vi "myRIO_BRig_RT_dataBlock_nRewards__L.vi"() -> (2 "output_nRewards__L":i32)   [LabVIEW 2014]
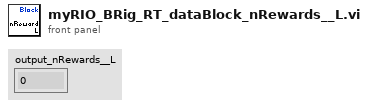
[diagram p1: front panel]
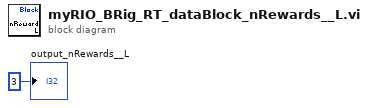
[diagram p0: block diagram]
diagram:
  "output_nRewards__L" <- 3 ("output_iBlock")
